vi "forLoop.vi"() -> ()   [LabVIEW 2021]
panel:
  out "Array 3":dbl[](array[numeric])
  in  "Array":dbl[](array[numeric])
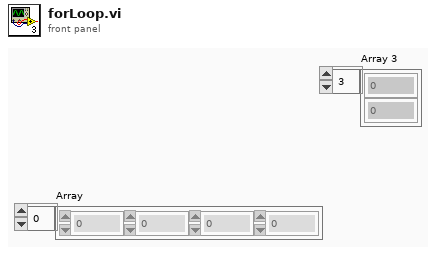
[diagram p1: front panel]
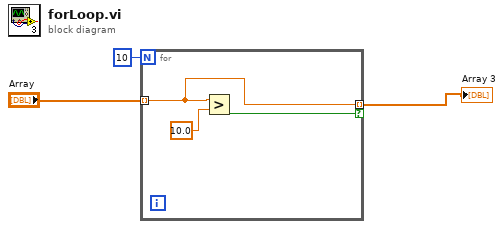
[diagram p0: block diagram]
diagram:
  n1 = for {
    N: 10 -> [_]
    tunnel: "Array" -> [w4] mode=indexing
    tunnel: [w4] -> w1 mode=indexing if=w5
    n2 = Greater?(x=w4, y=10.0) -> (0:w5:bool)
  }
  "Array 3" <- w1
